vi "relative_move_robust (SubVI).vi"(7 "deviceKey":string, 8 "error in (no error)":errorcluster, 9 "motor":i32, 10 "relativeSteps":i32, 11 ".NET Refnum in":refnum<k24>) -> (0 "error out":errorcluster, 3 ".NET Refnum out":refnum<k24>)   [LabVIEW 2018]
uses:
  C:/Users/yalem/GitHub/Documents/Optlev/LabView Code/Examples/Tilt Stage/CmdLib.dll
  Examples/Tilt Stage/CmdLib.dll
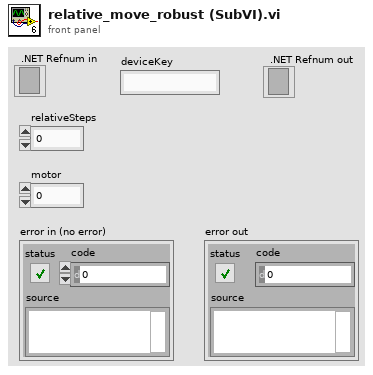
[diagram p1: front panel]
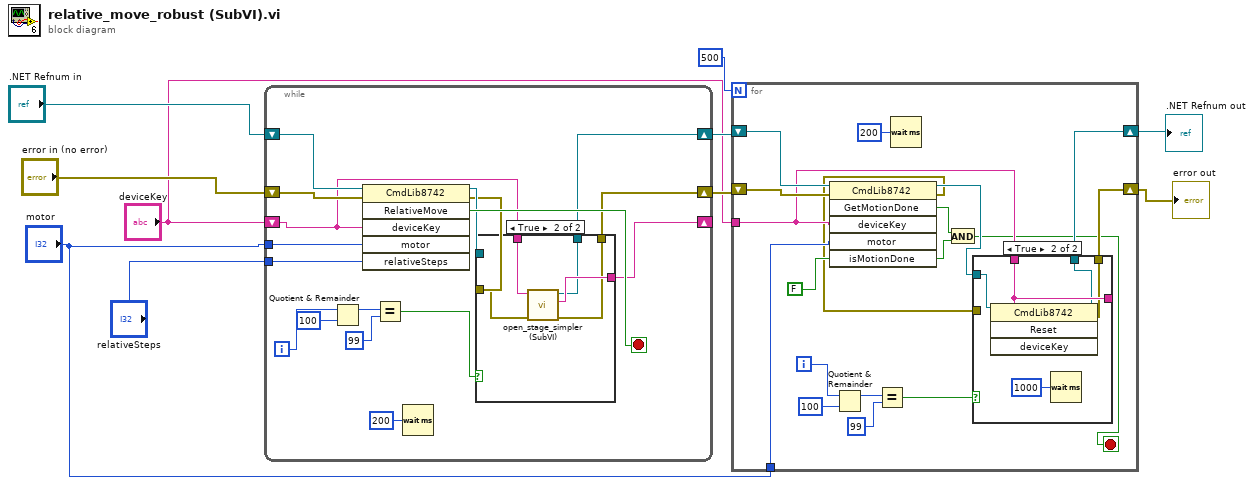
[diagram p0: block diagram]
diagram:
  n1 = while {
    tunnel: "motor" -> [w27]
    tunnel: "relativeSteps" -> [w25]
    shift-right: [w12] -> w6
    shift-left: "error in (no error)" -> [w26]
    shift-right: [w17] -> w7
    shift-left: ".NET Refnum in" -> [w24]
    shift-right: [w15] -> _
    shift-left: "deviceKey" -> [w16]
    i -> [w22]
    stop <- w23 stop-if-true
    n2 = Quotient & Remainder(x=w22, y=100) -> (x-y*floor(x/y)=w20:i32)  [unwired: 1 out]
    n3 = invoke class="CmdLib8742" method="RelativeMove"(reference=w24, error in=w26, "deviceKey"=w16, "motor"=w27, "relativeSteps"=w25) -> (reference out=w14:refnum<k24>, error out=w13:errorcluster, "RelativeMove"=w23:bool)  [unwired: 1 in, 3 out]
    n4 = Equal?(x=w20, y=99) -> (x = y?=w18:bool)
    n5 = Wait (ms)(milliseconds to wait=u32 200) -> ()  [unwired: 1 out]
    n6 = case shown="True" w18 {
      tunnel: [w30 w31] -> w17
      tunnel: w16 -> [w28 w35]
      tunnel: [w28 w34] -> w15
      tunnel: w14 -> [w30 _]
      tunnel: w13 -> [w29 w33]
      tunnel: [w29 w32] -> w12
      frame False {
      }
      frame True {
        n7 = call "open_stage_simpler (SubVI).vi"("error in (no error)"=w33, "IP address"=w35) -> ("error out"=w32:errorcluster, "deviceKey"=w34:string, "reference"=w31:refnum<k24>)  [unwired: 7 in]
      }
    }
  }
  n8 = for {
    N: 500 -> [_]
    shift-right: [w43] -> w2
    shift-left: w6 -> [w53]
    shift-right: [w42] -> w3
    shift-left: w7 -> [w52]
    tunnel: "deviceKey" -> [w46]
    tunnel: "motor" -> [w50]
    i -> [w38]
    stop <- w36 stop-if-true
    n9 = invoke class="CmdLib8742" method="GetMotionDone"(reference=w52, error in=w53, "deviceKey"=w46, "motor"=w50, "isMotionDone"=FALSE) -> (reference out=w45:refnum<k24>, error out=w44:errorcluster, "GetMotionDone"=w48:bool, "isMotionDone"=w47:bool)  [unwired: 1 in, 2 out]
    n10 = Quotient & Remainder(x=w38, y=100) -> (x-y*floor(x/y)=w40:i32)  [unwired: 1 out]
    n11 = Equal?(x=w40, y=99) -> (x = y?=w37:bool)
    n12 = Wait (ms)(milliseconds to wait=u32 200) -> ()  [unwired: 1 out]
    n13 = And(x=w48, y=w47) -> (x .and. y?=w36:bool)
    n14 = case shown="True" w37 {
      tunnel: [w56 w59] -> w42
      tunnel: w46 -> [w54 w60]
      tunnel: [w54 w60] -> _
      tunnel: w45 -> [w56 w61]
      tunnel: w44 -> [w55 _]
      tunnel: [w55 w58] -> w43
      frame False {
      }
      frame True {
        n15 = invoke class="CmdLib8742" method="Reset"(reference=w61, "deviceKey"=w60) -> (reference out=w59:refnum<k24>, error out=w58:errorcluster)  [unwired: 2 in, 2 out]
        n16 = Wait (ms)(milliseconds to wait=u32 1000) -> ()  [unwired: 1 out]
      }
    }
  }
  "error out" <- w2
  ".NET Refnum out" <- w3
